vi "文件对话框类型选择.vi"(8 "error in":errorcluster, 11 "Start Path":path=path "" caption="start path") -> (0 "error out":errorcluster, 1 "Exists?":bool caption="exists", 2 "Cancelled?":bool caption="cancelled", 3 "Selected File Path":path caption="selected path")   [LabVIEW 2009]
panel:
  in  "Filetype Patterns":T1(array[cluster])=[{"Pattern Label"="Recommended Image", "Patterns"=["*.png"]}, {"Pattern Label"="Lossless Image", "Patterns"=["*.png", "*.gif", "*.tif", "*.bmp"]}, {"Pattern Label"="Lossy Image", "Patterns"=["*.jpg"]}, {"Pattern Label"="Other Formats", "Patterns"=["*.pdf", "*.doc", "*.odg"]}]
  # "Inputs"
  # "Outputs"
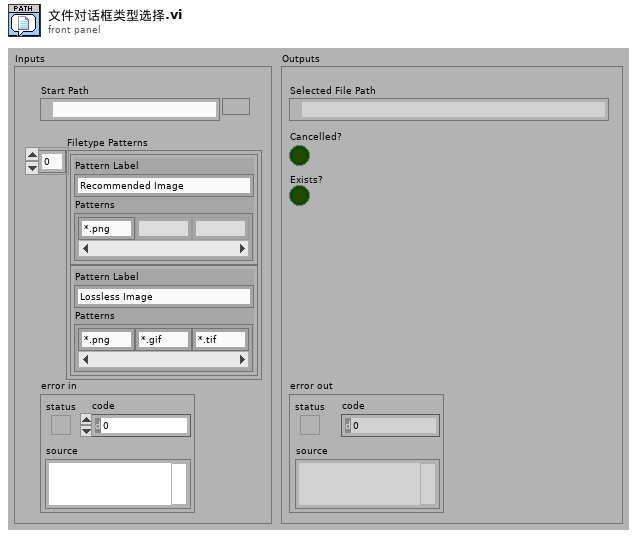
[diagram p1: front panel]
types:
  T1 = cluster{"Pattern Label":string, "Patterns":string[]}[]
  T2 = cluster{"Pattern Label":string, "Patterns":string[]}
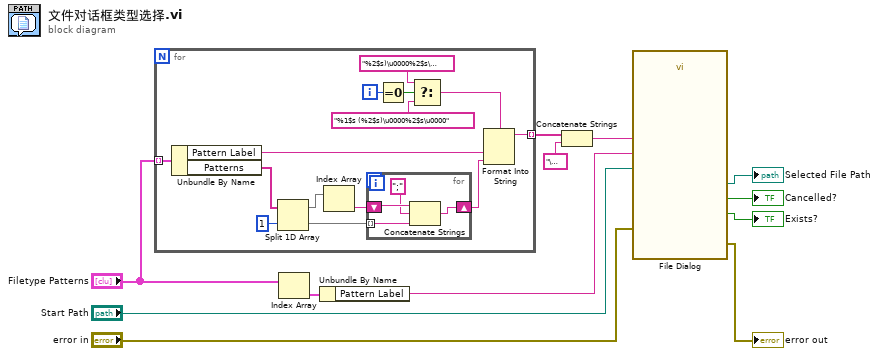
[diagram p0: block diagram]
diagram:
  n1 = for {
    tunnel: "Filetype Patterns" -> [w21] mode=indexing
    tunnel: [w19] -> w10 mode=indexing
    i -> [w26]
    n2 = Unbundle By Name(w21) -> ("Pattern Label"=w20:string, "Patterns"=w13:string[])
    n3 = Split 1D Array(array=w13, index=1) -> (first subarray=w17:string[], second subarray=w16:string[])
    n4 = Index Array(array=w17) -> (element=w18:string)  [unwired: 1 in]
    n5 = for {
      tunnel: w16 -> [w29] mode=indexing
      shift-right: [w27] -> w14
      shift-left: w18 -> [w30]
      n6 = Concatenate Strings(w30, ";" ("string"), w29) -> (w27:string)
    }
    n7 = Equal To 0?(x=w26) -> (x = 0?=w25:bool)
    n8 = Select(t="%2$s)\u0000%2$s\u0000" ("format string"), s=w25, f="%1$s (%2$s)\u0000%2$s\u0000" ("format string")) -> (s? t:f=w22:string)
    n9 = Format Into String(format string=w22, w20, w14) -> (resulting string=w19:string)  [unwired: 2 in, 1 out]
  }
  n10 = Index Array(array="Filetype Patterns") -> (element=w12:T2)  [unwired: 1 in]
  n11 = Unbundle By Name(w12) -> ("Pattern Label"=w8:string)
  n12 = Concatenate Strings(w10, "\u0000" ("format string")) -> (w9:string)
  n13 = call "File Dialog"("start path"="Start Path", "error in"="error in", "pattern (all files)"=w9, "pattern label"=w8) -> ("selected path"=→"Selected File Path":path, "exists"=→"Exists?":bool, "cancelled"=→"Cancelled?":bool, "error out"=→"error out":errorcluster)  [unwired: 3 in, 5 out]
